vi "LAN Config Link.vi"(0 "VISA resource name":refnum<visa-resource-name>, 5 "Node In":string, 7 "Autoconnect (On)":bool=TRUE, 9 "Link Timeout (s)":dbl=1.0, 11 "error in":errorcluster, 12 "Nagle (On)":bool=TRUE, 13 "LXI Domain (0)":u8) -> (4 "VISA resource name out":refnum<visa-resource-name>, 6 "Node Out":string, 14 "Command String":string, 15 "error out":errorcluster)   [LabVIEW 2013, in "Keithley 2600 Series.lvlib"]
doc: "This VI configures the instrument's LAN link settings.\n\nThis VI does not configure TCP/IP settings. Use LAN Config TCPIP.vi to configure TCP/IP settings.\n\n<b>Functions and Attributes Used</b>\nlan.autoconnect\nlan.config.autonegotiate\nlan.config.duplex\nlan.config.speed\nlan.linktimeout\nlan.lxidomain\nlan.nagle"
uses:
  Keithley 2600 Series.lvlib
  Private/GlobalVariables.vi
panel:
  # "(c) 2008 Keithley Instruments, Inc.  ALL RIGHTS RESERVED."
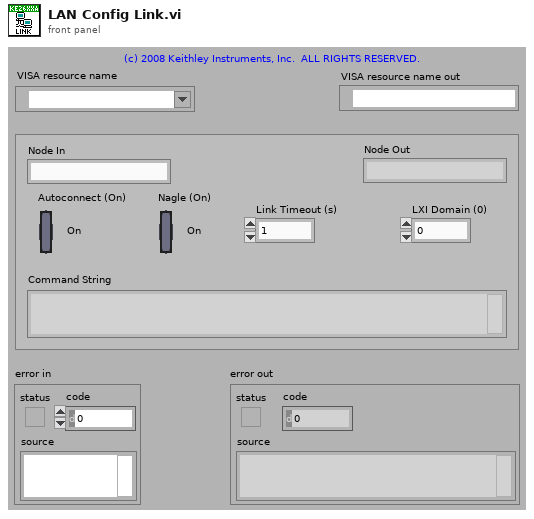
[diagram p1: front panel]
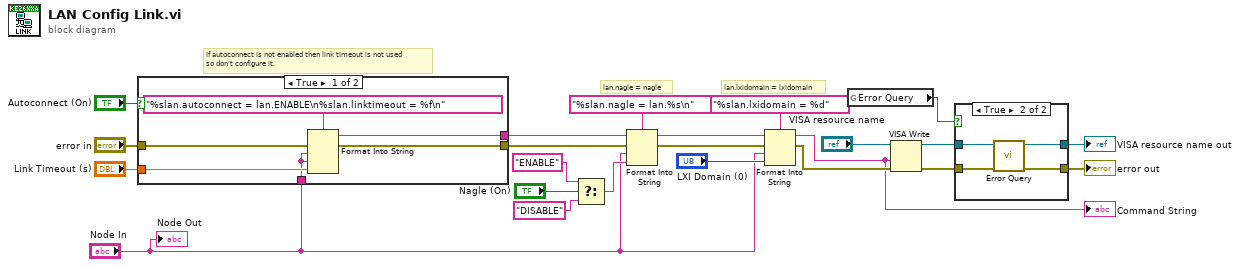
[diagram p0: block diagram]
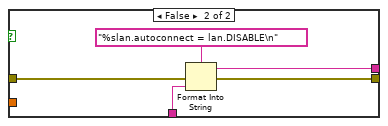
[diagram p3: hidden frame]
diagram:
  # "lan.lxidomain = lxidomain"
  # "lan.nagle = nagle"
  # "If autoconnect is not enabled then link timeout is not used\nso don't configure it."
  n1 = case shown="True" "Autoconnect (On)" {
    tunnel: "Link Timeout (s)" -> [w28 _]
    tunnel: "error in" -> [w27 w31]
    tunnel: [w26 w32] -> w2
    tunnel: [w25 w33] -> w3
    tunnel: "Node In" -> [w24 w30]
    frame True {
      n2 = Format Into String(format string="%slan.autoconnect = lan.ENABLE\n%slan.linktimeout = %f\n", error in=w27, w24, w24, w28) -> (resulting string=w25:string, error out=w26:errorcluster)  [unwired: 1 in]
    }
    frame False {
      n3 = Format Into String(format string="%slan.autoconnect = lan.DISABLE\n", error in=w31, w30) -> (resulting string=w33:string, error out=w32:errorcluster)  [unwired: 1 in]
    }
  }
  n4 = Select(t="ENABLE", s="Nagle (On)", f="DISABLE") -> (s? t:f=w16:string)
  n5 = Format Into String(format string="%slan.nagle = lan.%s\n", initial string=w3, error in=w2, "Node In", w16) -> (resulting string=w12:string, error out=w13:errorcluster)
  n6 = Format Into String(format string="%slan.lxidomain = %d", initial string=w12, error in=w13, "Node In", "LXI Domain (0)") -> (resulting string=w4:string, error out=w11:errorcluster)
  "Command String" <- w4
  n7 = global read "GlobalVariables.vi" "Error Query"() -> (w7:bool)
  n8 = VISA Write(VISA resource name="VISA resource name", write buffer=w4, error in (no error)=w11) -> (VISA resource name out=w9:refnum<visa-resource-name>, error out=w8:errorcluster)  [unwired: 1 out]
  n9 = case shown="True" w7 {
    tunnel: w9 -> [w36 w40]
    tunnel: w8 -> [w35 w39]
    tunnel: [w36 w38] -> w6
    tunnel: [w35 w37] -> w5
    frame False {
    }
    frame True {
      n10 = call "Error Query.vi"("error in (no error)"=w39, "VISA resource name"=w40) -> ("error out"=w37:errorcluster, "VISA resource name out"=w38:refnum<visa-resource-name>)  [unwired: 8 out]
    }
  }
  "VISA resource name out" <- w6
  "error out" <- w5
  "Node Out" <- "Node In"
